vi "Main_01b.vi"() -> ()   [LabVIEW 2020]
uses:
  2f0d15ab-f4ea-4645-b881-faf2cc17d9a1.vi
  <vilib>/Comparison/Less/Less Functor/Less Functor.lvclass
panel:
  out "reversed array":u32[](array[numeric])
  out "max value":u32
  in  "Input":string="3264\n4043\n2537\n3319\n2485\n3218\n5611\n1753\n7232\n3265\n1751\n2233\n\n10589\n5121\n11465\n9307\n1347\n9392\n12037\n\n6025\n4328\n3982\n4487\n1139\n1440\n2970\n3390\n1844\n5400\n1651\n4109\n3584\n2926\n4297\n\n8921\n13298\n12300\n5607\n3304\n5037\n\n1729\n10057\n\n3538\n3984\n3451\n5638\n2880\n1008\n2940\n6245\n3865\n5060\n2878\n2460\n6557\n\n1584\n6391\n3479\n2264\n2683\n3680\n1183\n5121\n6499\n5543\n1192\n4818\n\n1337\n8128\n8966\n7601\n7749\n5017\n3251\n1074\n6095\n\n11824\n17144\n5396\n15416\n\n6244\n6589\n4953\n4250\n1422\n1252\n4555\n5240\n4244\n4088\n\n27353\n\n6629\n7231\n7673\n7029\n6994\n6347\n6381\n1503\n2145\n1114\n6068\n\n3473\n3935\n4054\n3558\n3818\n5370\n4807\n2703\n5407\n2532\n6833\n1675\n\n20016\n7..."
  # "--- Day 1: Calorie Counting ---\nSanta's reindeer typically eat regular reindeer food, but they need a lot of magical energy to deliver presents on Christmas. For that, their favorite snack is a special type of star fruit that only grows deep in the jungle. The Elves have brought you on their annual expedition to the grove where the fruit grows.\n\nTo supply enough magical energy, the expedition needs to retrieve a minimum of fifty stars by December 25th. Although the Elves assure you that the grove has plenty of fruit, you decide to grab any fruit you see along the way, just in case.\n\nCollect stars by solving puzzles. Two puzzles will be made available on each day in the Advent calendar; the second puzzle is unlocked when you complete the first. Each puzzle grants one star. Good luck!\n\nThe jungle must be too overgrown and difficult to navigate in vehicles or access from the air; the Elves' expedition traditionally goes on foot. As your boats approach land, the Elves begin taking inventory of their supplies. One important consideration is food - in particular, the number of Calories each Elf is carrying (your puzzle input).\n\nThe Elves take turns writing down the number of Calories contained by the various meals, snacks, rations, etc. that they've brought with them, one item per line. Each Elf separates their own inventory from the previous Elf's inventory (if any) by a blank line.\n\nFor example, suppose the Elves finish writing their items' Calories and end up with the following list:\n\n1000\n2000\n3000\n\n4000\n\n5000\n6000\n\n7000\n8000\n9000\n\n10000\nThis list represents the Calories of the food carried by five Elves:\n\nThe first Elf is carrying food with 1000, 2000, and 3000 Calories, a total of 6000 Calories.\nThe second Elf is carrying one food item with 4000 Calories.\nThe third Elf is carrying food with 5000 and 6000 Calories, a total of 11000 Calories.\nThe fourth Elf is carrying food with 7000, 8000, and 9000 Calories, a total of 24000 Calories.\nThe fifth Elf is carrying one food item with 10000 Calories.\nIn case the Elves get hungry and need extra snacks, they need to know which Elf to ask: they'd like to know how many Calories are being carried by the Elf carrying the most Calories. In the example above, this is 24000 (carried by the fourth Elf).\n\nFind the Elf carrying the most Calories. How many total Calories is that Elf carrying?\n\nYour puzzle answer was 72070.\n\n--- Part Two ---\nBy the time you calculate the answer to the Elves' question, they've already realized that the Elf carrying the most Calories of food might eventually run out of snacks.\n\nTo avoid this unacceptable situation, the Elves would instead like to know the total Calories carried by the top three Elves carrying the most Calories. That way, even if one of those Elves runs out of snacks, they still have two backups.\n\nIn the example above, the top three Elves are the fourth Elf (with 24000 Calories), then the third Elf (with 11000 Calories), then the fifth Elf (with 10000 Calories). The sum of the Calories carried by these three elves is 45000.\n\nFind the top three Elves carrying the most Calories. How many Calories are those Elves carrying in total?\n\nYour puzzle answer was 211805."
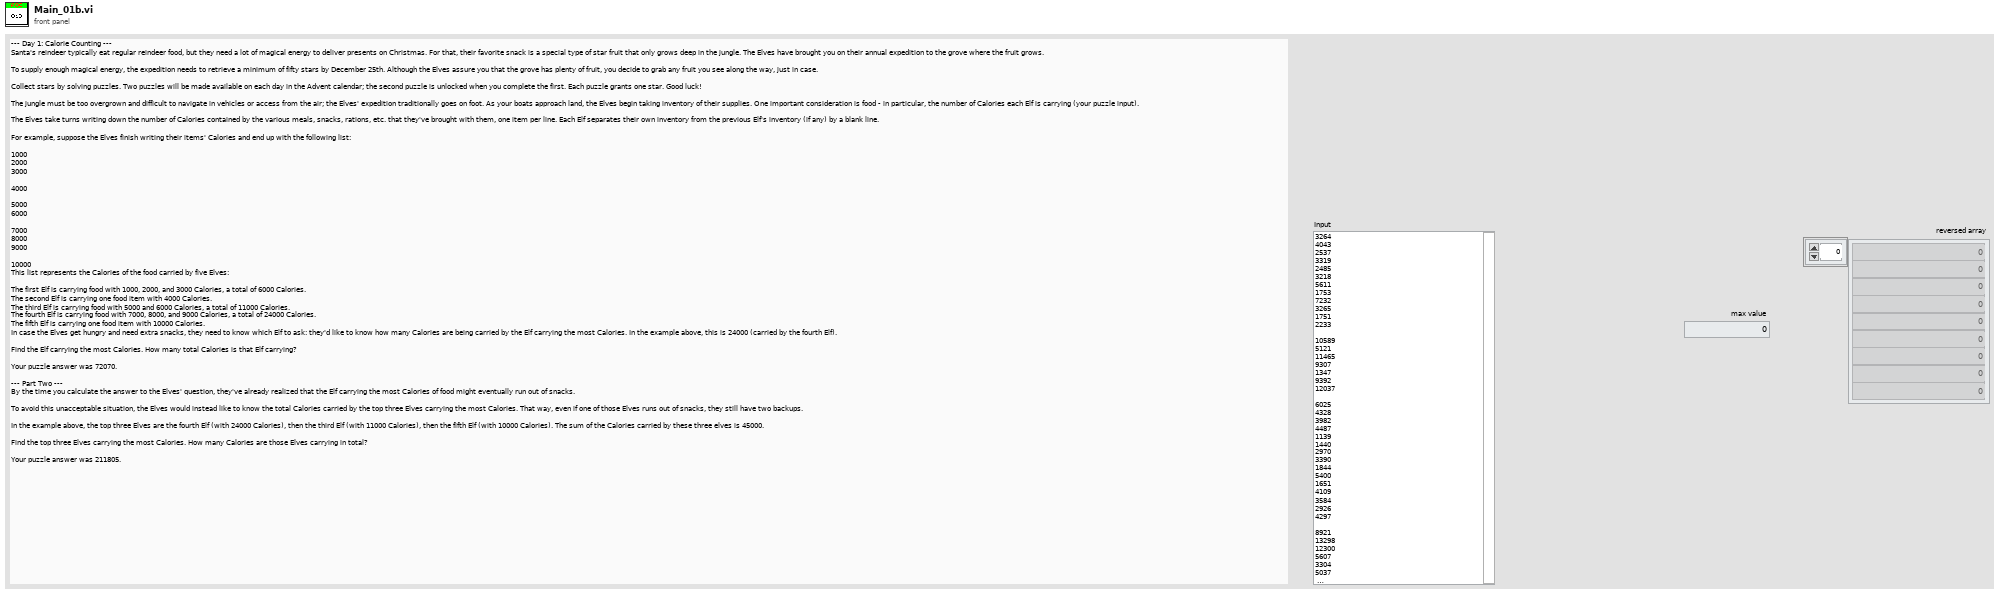
[diagram p1: front panel]
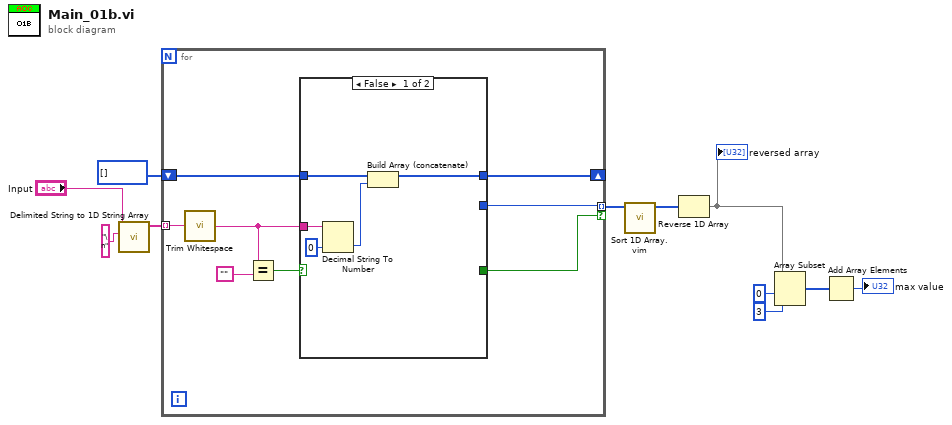
[diagram p0: block diagram]
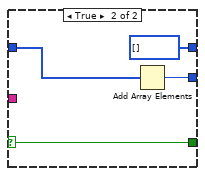
[diagram p2: hidden frame]
diagram:
  n1 = call <vilib>:"Delimited String to 1D String Array.vi"("delimiter"="\n", "delimited string"="Input") -> ("string array"=w9:string[])  [unwired: 9 in]
  n2 = for {
    tunnel: w9 -> [w19] mode=indexing
    shift-right: [w14] -> _
    shift-left: u32[] [] ("trimmed string") -> [w17]
    tunnel: [w13] -> w7 mode=indexing if=w12
    n3 = call <vilib>:"Trim Whitespace.vi"("string"=w19) -> ("trimmed string"=w15:string)  [unwired: 1 in]
    n4 = Equal?(x=w15, y="") -> (x = y?=w16:bool)
    n5 = case shown="False" w16 {
      selector: w16 -> [_ w25]
      tunnel: w17 -> [w24 w26]
      tunnel: w15 -> [w22 _]
      tunnel: [w23 u32[] []] -> w14
      tunnel: [_ w27] -> w13
      tunnel: [_ w25] -> w12
      frame False {
        n6 = Decimal String To Number(string=w22, default (0L)=u32 0 ("default (0 I32)")) -> (number=w21:u32)  [unwired: 1 in, 1 out]
        n7 = Build Array (concatenate)(w24, w21) -> (w23:u32[])
      }
      frame True {
        n8 = Add Array Elements(numeric array=w26) -> (sum=w27:u32)
      }
    }
  }
  n9 = call "Sort 1D Array.vim"("unsorted array"=w7) -> ("sorted array"=w6:u32[])  [unwired: 10 in]
  n10 = Reverse 1D Array(array=w6) -> (reversed array=w5:u32[])
  "reversed array" <- w5
  n11 = Array Subset(array=w5, index=0, length=3) -> (w2:u32[])
  n12 = Add Array Elements(numeric array=w2) -> (sum=→"max value":u32)
